vi "Validate.vi"(8 "error in (no error)":errorcluster, 11 "Build in":refnum<class "AB_RESTfulWebService.lvclass">) -> (0 "error out":errorcluster, 3 "Build out":refnum<class "AB_RESTfulWebService.lvclass">)   [LabVIEW 2020, in "AB_RESTfulWebService.lvclass"]
uses:
  <vilib>/AppBuilder/AB_Classes/RESTful/AB_RESTfulWebService.lvclass
  e:/builds/penguin/labview/branches/2020/dev/dist/vi.lib/AppBuilder/AB_Classes/Build/AB_Build.lvclass
  <vilib>/AppBuilder/AB_Classes/RESTful/AB_RESTfulWebService.lvclass/AB_RESTfulWebService.ctl
  <resource>/Framework/Providers/Common/provcom_StringGlobals.vi
  <vilib>/AppBuilder/AB_Classes/WebService/AB_WebService.lvclass
  <vilib>/AppBuilder/AB_Classes/Build/AB_Build.lvclass
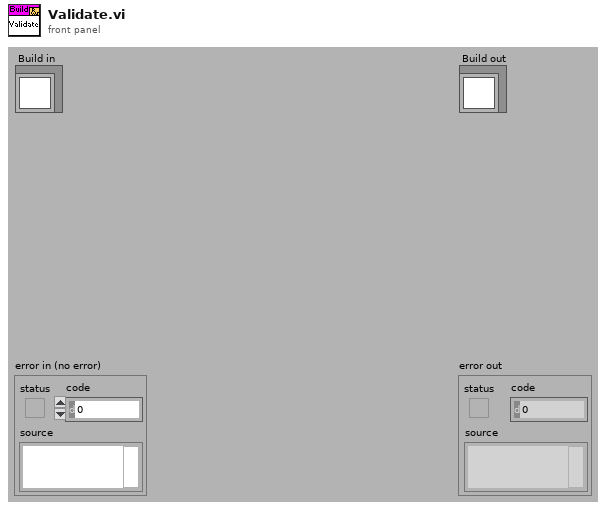
[diagram p1: front panel]
types:
  T1 = typedef "AB_RESTfulWebService.ctl" = cluster{"routing templates":T2[], "defaultStaticDoc":string, "eng_attributes":T5[], "Privilege Mapping":cluster{"Privilege":string, "Description":string, "Role":string}[]}
  T2 = typedef "AB_RESTful_RoutingTemplate.ctl" = cluster{"Template":string, "Routing Type":T3, "HTTP Method Type":T4, "VIName":string, "Default String":string, "Require API key":bool, "Auth permissions":string[], "eng_Static Alias":string, "Required Privilege":string}
  T3 = typedef "AB_RESTful_RoutingType.ctl" = enum32{"Method", "Static"}
  T4 = typedef "AB_RESTful_HTTPMethodType.ctl" = enum32{"GET", "POST", "PUT", "DELETE"}
  T5 = typedef "AB_RESTful_ServiceAttribute.ctl" = cluster{"Name":string, "Service Attribute Type":T6, "Value":string}
  T6 = typedef "AB_RESTful_ServiceAttributeType.ctl" = enum32{"String", "Path"}
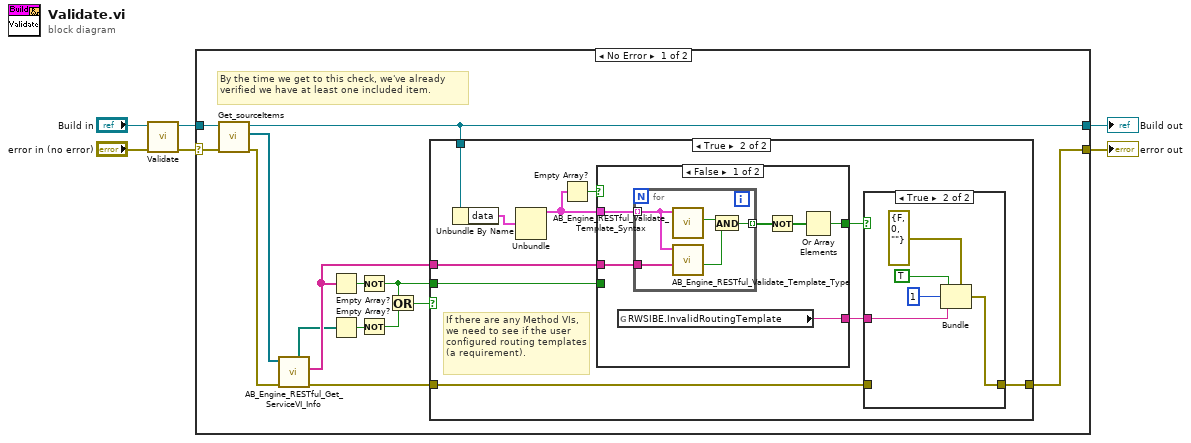
[diagram p0: block diagram]
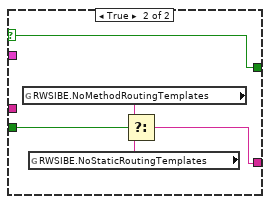
[diagram p3: hidden frame]
diagram:
  n1 = call-parent "Validate.vi"("error in (no error)"="error in (no error)", "Build in"="Build in") -> ("error out"=w4:errorcluster, "Build out"=w3:refnum<class "AB_RESTfulWebService.lvclass">)  [unwired: 8 in]
  n2 = case shown="No Error" w4 {
    selector: w4 -> [w18 w54]
    tunnel: w3 -> [w19 w55]
    tunnel: [w14 w55] -> w2
    tunnel: [w20 w54] -> w1
    frame No Error {
      # "By the time we get to this check, we've already verified we have at least one included item."
      n3 = call <vilib>:"Get_sourceItems.vi"("error in (no error)"=w18, "Class in"=w19) -> ("error out"=w16:errorcluster, "sourceItems"=w17:refnum<class "AB_Source.lvclass">[], "Class out"=w14:refnum<class "AB_RESTfulWebService.lvclass">)  [unwired: 7 in]
      n4 = call <vilib>:"AB_Engine_RESTful_Get_ServiceVI_Info.vi"("error in (no error)"=w16, "sourceItems"=w17) -> ("error out"=w15:errorcluster, "MethodVI  names"=w13:string[], "IncludedFile paths"=w12:path[])  [unwired: 5 in, 2 out]
      n5 = Empty Array?(array=w13) -> (empty?=w10:bool)
      n6 = Empty Array?(array=w12) -> (empty?=w11:bool)
      n7 = Not(x=w10) -> (.not. x?=w7:bool)
      n8 = Not(x=w11) -> (.not. x?=w8:bool)
      n9 = Or(x=w7, y=w8) -> (x .or. y?=w9:bool)
      n10 = case shown="True" w9 {
        tunnel: [w21 w31] -> w20
        tunnel: w15 -> [w21 w30]
        tunnel: w14 -> [_ w29]
        tunnel: w13 -> [_ w23]
        tunnel: w7 -> [_ w22]
        frame False {
          # "If there are no method VIs, then the user must have configured only Aux VIs. Nothing more to check."
        }
        frame True {
          # "If there are any Method VIs, we need to see if the user configured routing templates (a requirement)."
          n11 = Unbundle By Name(w29) -> ("data"=w27:T1)
          n12 = Unbundle(w27) -> ("routing templates"=w26:T2[])  [unwired: 3 out]
          n13 = Empty Array?(array=w26) -> (empty?=w28:bool)
          n14 = case shown="False" w28 {
            selector: w28 -> [_ w47]
            tunnel: w23 -> [w37 _]
            tunnel: w26 -> [w36 _]
            tunnel: [w34 w47] -> w25
            tunnel: [w33 w44] -> w24
            tunnel: w22 -> [_ w46]
            frame False {
              n15 = global read "provcom_StringGlobals.vi" "RWSIBE.InvalidRoutingTemplate"() -> (w33:string)
              n16 = for {
                tunnel: w37 -> [w42]
                tunnel: w36 -> [w39] mode=indexing
                tunnel: [w41] -> w32 mode=indexing
                n17 = call <vilib>:"AB_Engine_RESTful_Validate_Template_Syntax.vi"("RESTful VI routing template in"=w39) -> ("valid syntax"=w38:bool)  [unwired: 10 in]
                n18 = call <vilib>:"AB_Engine_RESTful_Validate_Template_Type.vi"("source file names"=w42, "RESTful VI routing template in"=w39) -> ("template type vald"=w40:bool)  [unwired: 8 in, 1 out]
                n19 = And(x=w38, y=w40) -> (x .and. y?=w41:bool)
              }
              n20 = Not(x=w32) -> (.not. x?=w35:bool[])
              n21 = Or Array Elements(Boolean array=w35) -> (logical OR=w34:bool)
            }
            frame True {
              n22 = global read "provcom_StringGlobals.vi" "RWSIBE.NoMethodRoutingTemplates"() -> (w45:string)
              n23 = global read "provcom_StringGlobals.vi" "RWSIBE.NoStaticRoutingTemplates"() -> (w43:string)
              n24 = Select(t=w45, s=w46, f=w43) -> (s? t:f=w44:string)
            }
          }
          n25 = case shown="True" w25 {
            tunnel: [w48 w50] -> w31
            tunnel: w30 -> [w48 _]
            tunnel: w24 -> [_ w49]
            frame False {
            }
            frame True {
              n26 = Bundle(cluster=errorcluster {"status"=FALSE, "code"=0, "source"=""} ("error IO"), "status"=TRUE, "code"=1, "source"=w49) -> (w50:errorcluster)
            }
          }
        }
      }
    }
    frame Error {
    }
  }
  "error out" <- w1
  "Build out" <- w2
